vi "tester.vi"() -> ()   [LabVIEW 2018]
uses:
  <vilib>/Utility/file.llb/Read Delimited Spreadsheet (DBL).vi
  build/bin/RCVAnalysis.dll
panel:
  out "FWHM":dbl[](array[numeric])
  out "fullHeight":dbl[](array[numeric])
  out "xValsHalfHeight":dbl[][](array[numeric])
  out "peakArea":dbl[](array[numeric])
  out "xValsFullHeight":dbl[][](array[numeric])
  out "indexes":i32[](array[numeric])
  out "locations":dbl[](array[numeric])
  out "size(s)":i32
  out "heights":dbl[](array[numeric])
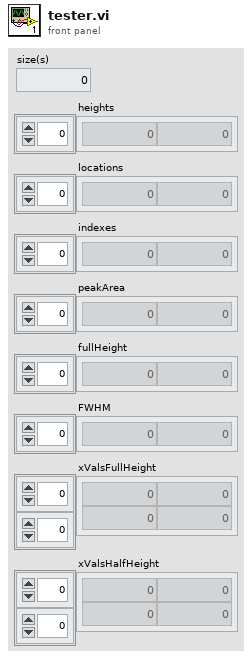
[diagram p1: front panel]
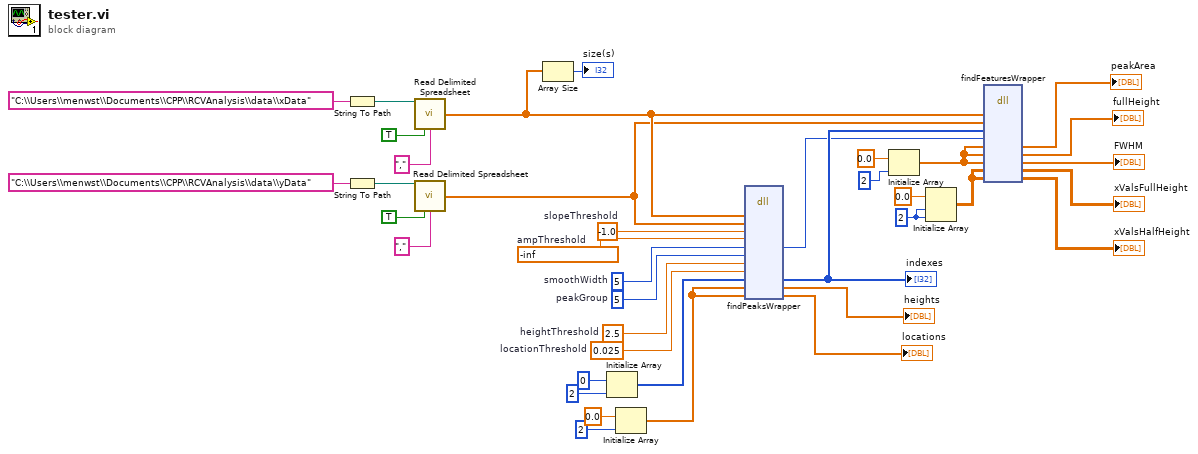
[diagram p0: block diagram]
diagram:
  w7 = 2 ("xnumRows")
  w23 = -inf  # ampThreshold
  w21 = 0.025  # locationThreshold
  w22 = 2.5  # heightThreshold
  w26 = 5  # peakGroup
  w25 = u32 5  # smoothWidth
  w24 = -1.0  # slopeThreshold
  n1 = String To Path(string="C:\\Users\\menwst\\Documents\\CPP\\RCVAnalysis\\data\\xData") -> (path=w34:path)
  n2 = String To Path(string="C:\\Users\\menwst\\Documents\\CPP\\RCVAnalysis\\data\\yData") -> (path=w35:path)
  n3 = call-poly <vilib>:"Read Delimited Spreadsheet.vi"("file path (dialog if empty)"=w34, "transpose? (F)"=TRUE, "delimiter (\\t)"="," ("delimiter (\\t)")) -> ("first row"=w14:dbl[])  [unwired: 7 in, 5 out]
  n4 = call-poly <vilib>:"Read Delimited Spreadsheet.vi"("file path (dialog if empty)"=w35, "transpose? (F)"=TRUE, "delimiter (\\t)"="," ("delimiter (\\t)")) -> ("first row"=w13:dbl[])  [unwired: 7 in, 5 out]
  n5 = Array Size(array=w14) -> (size(s)=→"size(s)":i32)
  n6 = Initialize Array(0 ("dimension size"), 2 ("dimension size")) -> (w18:i32[])
  n7 = Initialize Array(0.0 ("element"), 2 ("dimension size")) -> (w10:dbl[])
  n8 = dll-call lib="C:/Users/menwst/Documents/CPP/RCVAnalysis/build/bin/RCVAnalysis.dll" fn="findPeaksWrapper"("xdata"=w14, "ydata"=w13, "slopeThreshold"=w24, "ampThreshold"=w23, "smoothWidth"=w25, "peakGroup"=w26, "heightThreshold"=w22, "locationThreshold"=w21, "indexes"=w18, "heights"=w10, "locations"=w10) -> ("smoothWidth"=w11:u32, "indexes"=w12:i32[], "heights"=→"heights":dbl[], "locations"=→"locations":dbl[])  [unwired: 11 in, 2 out]
  "indexes" <- w12
  n9 = Initialize Array(0.0 ("element"), 2 ("xnumRows")) -> (w9:dbl[])
  n10 = Initialize Array(0.0 ("element"), w7, w7) -> (w6:dbl[][])
  n11 = dll-call lib="C:/Users/menwst/Documents/CPP/RCVAnalysis/build/bin/RCVAnalysis.dll" fn="findFeaturesWrapper"("xdata"=w14, "ydata"=w13, "indexes"=w12, "smoothWidth"=w11, "peakArea"=w9, "fullHeight"=w9, "FWHM"=w9, "xValsFullHeight"=w6, "xValsHalfHeight"=w6) -> ("peakArea"=→"peakArea":dbl[], "fullHeight"=→"fullHeight":dbl[], "FWHM"=→"FWHM":dbl[], "xValsFullHeight"=→"xValsFullHeight":dbl[][], "xValsHalfHeight"=→"xValsHalfHeight":dbl[][])  [unwired: 8 in, 2 out]
